vi "ServicePushState.vi"(8 "error in (no error)":errorcluster, 10 "Cluster in":T2, 11 "Enum in":T1) -> (0 "error out":errorcluster, 2 "Cluster out":T2, 3 "Enum out":T1)   [LabVIEW 2018]
uses:
  Type_Def/Type_Def Actuator Controls.ctl
  Type_Def/Type_Def ControlState.ctl
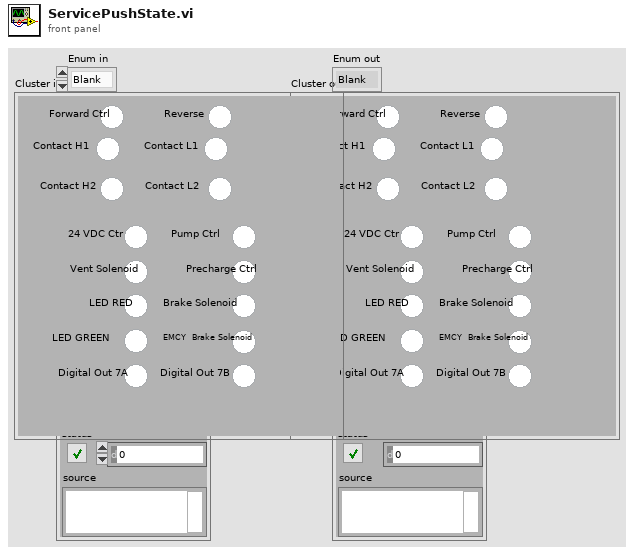
[diagram p1: front panel]
types:
  T1 = typedef "Type_Def ControlState.ctl" = enum16{"Blank", "Systems Check", "Idle", "Ready", "Pushing", "CrawlingPrecharge", "Braking", "Fault", "Boot Up", "Crawling", "Shutdown", "Service Push", "Service Wait", "Vent", "Precharge"}
  T2 = typedef "Type_Def Actuator Controls.ctl" = cluster{"Reverse ":bool, "Precharge Ctrl":bool, "Pump Ctrl":bool, "24 VDC Ctr":bool, "Vent Solenoid":bool, "Brake Solenoid":bool, "EMCY  Brake Solenoid":bool, "Digital Out 7B ":bool, "Forward Ctrl":bool, " Contact H2":bool, "Contact L2":bool, "LED RED":bool, "LED GREEN":bool, " Digital Out 7A":bool, " Contact H1":bool, "Contact L1":bool}
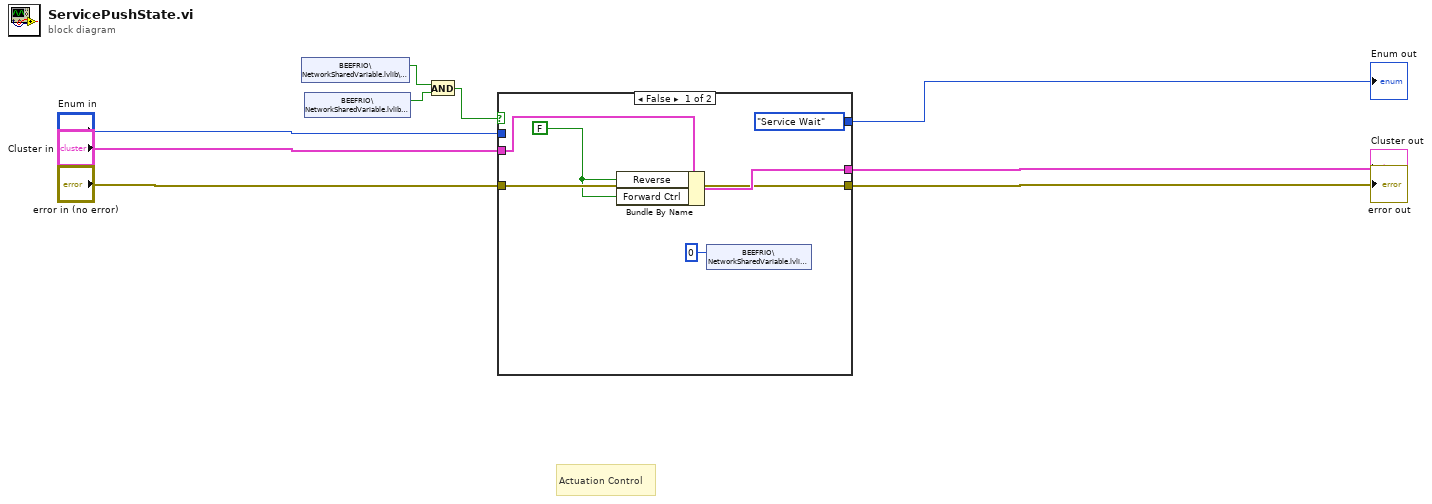
[diagram p0: block diagram]
diagram:
  # "Actuation Control"
  n1 = shared-variable "BEEFRIO\\NetworkSharedVariable.lvlib\\ServicePush"() -> (w2:bool)  [unwired: 1 in, 1 out]
  n2 = shared-variable "BEEFRIO\\NetworkSharedVariable.lvlib\\driveEnable"() -> (w1:bool)  [unwired: 1 in, 1 out]
  n3 = And(x=w2, y=w1) -> (x .and. y?=w3:bool)
  n4 = case shown="False" w3 {
    tunnel: "Enum in" -> [_ w18]
    tunnel: [Type_Def_ControlState."Service Wait" w18] -> w5
    tunnel: "Cluster in" -> [w12 w17]
    tunnel: [w14 w17] -> w7
    tunnel: [w13 w16] -> w8
    tunnel: "error in (no error)" -> [w13 w16]
    frame False {
      w10 = FALSE ("Digital Out 5")
      n5 = Bundle By Name(cluster=w12, "Reverse"=w10, "Forward Ctrl"=w10) -> (w14:T2)
      n6 = shared-variable "BEEFRIO\\NetworkSharedVariable.lvlib\\driveTarget"(i16 0 ("driveTarget")) -> ()  [unwired: 1 in, 1 out]
    }
    frame True {
    }
  }
  "error out" <- w8
  "Cluster out" <- w7
  "Enum out" <- w5
